vi "comand.vi"(8 "Param 2":string, 9 "Param 1":string, 10 "Serial device Brand":T1, 11 "Command":T2) -> (3 "Command to send":string)   [LabVIEW 2019, in "Serial Device.lvclass"]
uses:
  Serial Device.lvclass
  COMANDO.ctl
  Control 14.ctl
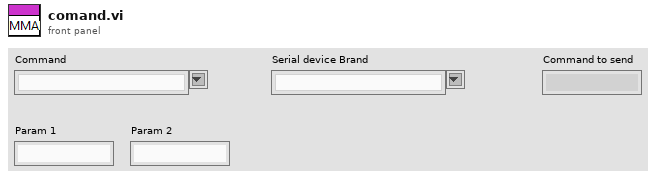
[diagram p1: front panel]
types:
  T1 = typedef "Serial Device.lvclass/Control 14.ctl" = string
  T2 = typedef "Serial Device.lvclass/COMANDO.ctl" = string
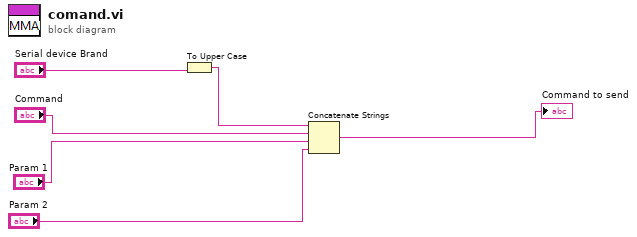
[diagram p0: block diagram]
diagram:
  n1 = To Upper Case(1:"Serial device Brand") -> (0:w5:T1)
  n2 = Concatenate Strings(w5, "Command", "Param 1", "Param 2") -> (→"Command to send":string)
